vi "Simulate Waveform in chart (Using DAC).vi"() -> ()   [LabVIEW 2020]
uses:
  <vilib>/DAQmx/read.llb/DAQmx Read (Analog 1D DBL 1Chan NSamp).vi
  <vilib>/DAQmx/create/channels.llb/DAQmx Create Channel (AI-Voltage-Basic).vi
  <vilib>/DAQmx/miscellaneous.llb/DAQmx Fill In Error Info.vi
panel:
  out "Waveform Chart":dbl[](graph)
  in  "stop 2":bool
  out "error out 2":errorcluster
  # "Simulate Waveform in Chart (Using DAC)"
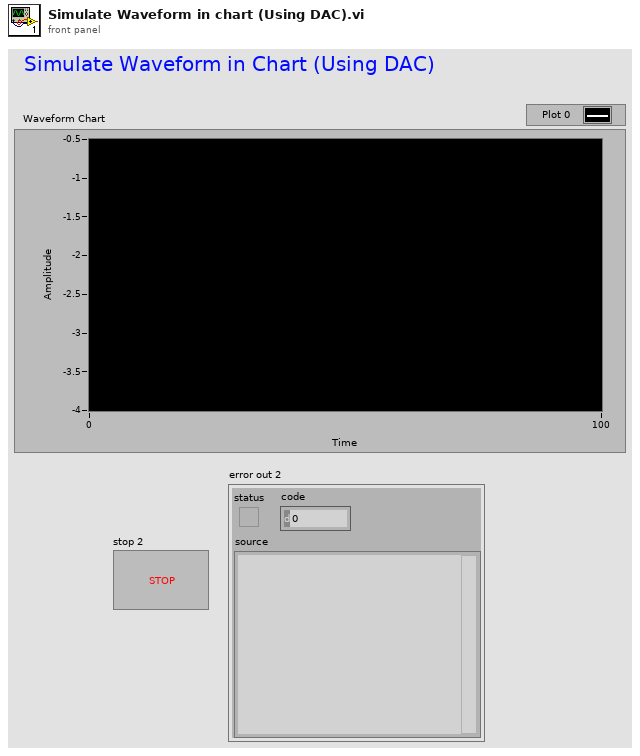
[diagram p1: front panel]
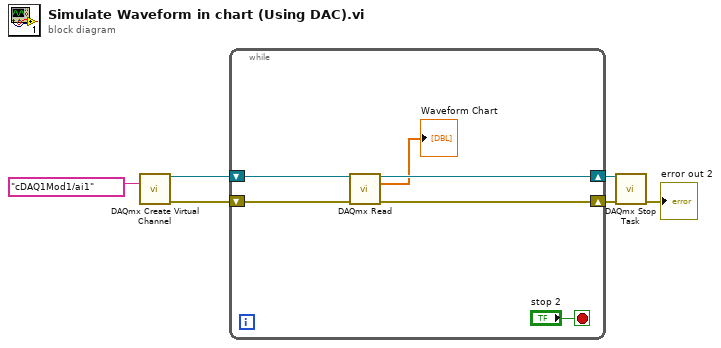
[diagram p0: block diagram]
diagram:
  n1 = call-poly <vilib>:"DAQmx Create Virtual Channel.vi"("physical channels"=tag "cDAQ1Mod1/ai1") -> ("task out"=w1:refnum<k21>, "error out"=w2:errorcluster)  [unwired: 13 in]
  n2 = while {
    shift-right: [w9] -> w3
    shift-left: w1 -> [w11]
    shift-right: [w8] -> w4
    shift-left: w2 -> [w10]
    stop <- "stop 2" stop-if-true
    n3 = call-poly <vilib>:"DAQmx Read.vi"("task/channels in"=w11, "error in"=w10) -> ("task out"=w9:refnum<k21>, "data"=→"Waveform Chart":dbl[], "error out"=w8:errorcluster)  [unwired: 11 in]
  }
  n4 = call <vilib>:"DAQmx Stop Task.vi"("task/channels in"=w3, "error in"=w4) -> ("error out"=→"error out 2":errorcluster)  [unwired: 12 in, 1 out]
